vi "Swap Panel Up.vi"(8 "error in (no error)":errorcluster, 10 "Panel":refnum<class "Panel.lvclass">, 11 "PanelArray in":refnum<class "PanelArray.lvclass">) -> (0 "error out":errorcluster, 3 "PanelArray out":refnum<class "PanelArray.lvclass">)   [LabVIEW 2018, in "OOPanel.lvlib" / "PanelArray.lvclass"]
uses:
  PanelArray.lvclass
  Panel/Panel.lvclass
  PanelArray.lvclass/PanelArray.ctl
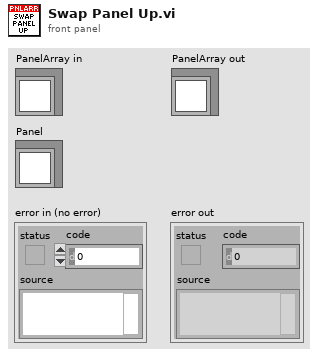
[diagram p1: front panel]
types:
  T1 = typedef "OOPanel.lvlib/PanelArray.lvclass/Ref Data.ctl" = cluster{"State":T2, "Refs":T3, "Events":T4, "Scrolling":T5, "Panels":T6}
  T2 = typedef "OOPanel.lvlib/PanelArray.lvclass/State.ctl" = cluster{"Defer Updates":bool, "Running":bool, "Dynamic Sizing":bool, "Borders":bool}
  T3 = typedef "OOPanel.lvlib/PanelArray.lvclass/Refs.ctl" = cluster{"SubPanels":refnum<vi>[], "Scrollbar":refnum<vi>, "Owning Panel":refnum<vi>}
  T4 = typedef "OOPanel.lvlib/PanelArray.lvclass/Events.ctl" = cluster{"Close":refnum<user-event>}
  T5 = typedef "OOPanel.lvlib/PanelArray.lvclass/Scrolling.ctl" = cluster{"Size":i32, "Max":i32, "Current":i32, "Top Index":i32, "Heights":i32[]}
  T6 = typedef "OOPanel.lvlib/PanelArray.lvclass/Panels.ctl" = cluster{"All":refnum<class "Panel.lvclass">[], "Visible":refnum<class "Panel.lvclass">[], "Blank":refnum<class "ArrayBlank.lvclass">}
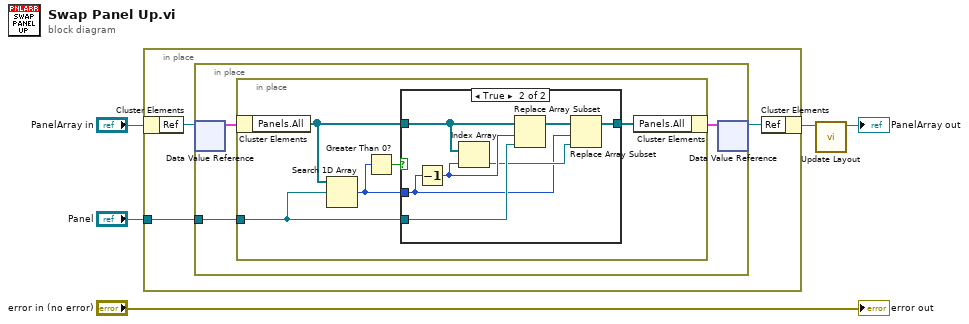
[diagram p0: block diagram]
diagram:
  n1 = in-place {
    in-place-border: "Panel" -> [w8]
    n2 = in-place-cluster #1("PanelArray in") -> ("Ref"=w7:refnum<data-value>)
    n3 = in-place {
      in-place-border: w8 -> [w9]
      n4 = in-place-dvr #2(w7) -> (w11:T1)  [unwired: 1 out]
      n5 = in-place {
        in-place-border: w9 -> [w12]
        n6 = in-place-cluster #3(w11) -> ("Panels.All"=w14:refnum<class "Panel.lvclass">[])
        n7 = Search 1D Array(1D array=w14, element=w12) -> (index of element=w15:i32)  [unwired: 1 in]
        n8 = Greater Than 0?(x=w15) -> (x > 0?=w16:bool)
        n9 = case shown="True" w16 {
          tunnel: w15 -> [_ w19]
          tunnel: w14 -> [w17 w24]
          tunnel: [w17 w18] -> w13
          tunnel: w12 -> [_ w23]
          frame False {
          }
          frame True {
            n10 = Decrement(x=w19) -> (x-1=w22:i32)
            n11 = Index Array(array=w24, index=w22) -> (element=w20:refnum<class "Panel.lvclass">)
            n12 = Replace Array Subset(array=w24, new element=w23, index=w22) -> (w21:refnum<class "Panel.lvclass">[])
            n13 = Replace Array Subset(array=w21, new element=w20, index=w19) -> (w18:refnum<class "Panel.lvclass">[])
          }
        }
        n14 = in-place-cluster #3("Panels.All"=w13) -> (w10:T1)
      }
      n15 = in-place-dvr #2(w10) -> (w6:refnum<data-value>)  [unwired: 1 out]
    }
    n16 = in-place-cluster #1("Ref"=w6) -> (w2:refnum<class "PanelArray.lvclass">)
  }
  n17 = call "Update Layout.vi"("PanelArray in"=w2) -> ("PanelArray out"=→"PanelArray out":refnum<class "PanelArray.lvclass">)  [unwired: 9 in, 1 out]
  "error out" <- "error in (no error)"
